vi "Set and Get Cell ItemName.vi"(6 "Cell":T1 caption="活动单元格:活动单元格", 7 "Mode":T2, 8 "错误输入":errorcluster, 10 "Item In":string, 11 "Mlistbox Ref":refnum<vi>) -> (0 "错误输出":errorcluster, 2 "Item Out":string, 3 "Mlistbox Ref Dup":refnum<vi>)   [LabVIEW 2012, in "Mlistbox Tools.lvlib"]
uses:
  Mlistbox Tools.lvlib
  ListBox/Custom Type/Read and Write Mode.ctl
  <vilib>/Utility/miscctls.llb/LVRowAndColumnTypeDef.ctl
  Set and Get ItemNames.vi
  ListBox/Listbox Tool.lvlib
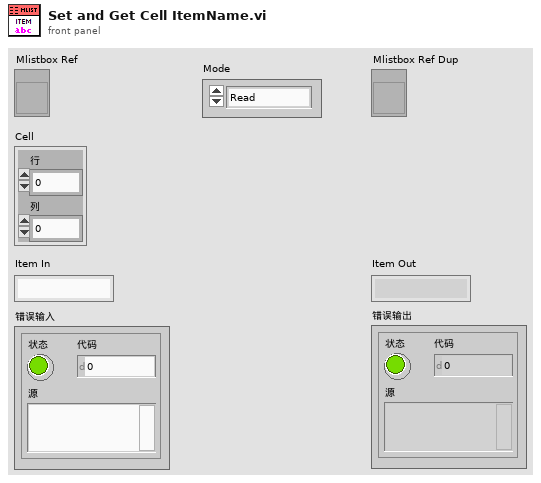
[diagram p1: front panel]
types:
  T1 = typedef "LVRowAndColumnTypeDef.ctl" = cluster{"Row":i32, "Column":i32}
  T2 = typedef "Listbox Tool.lvlib/Read and Write Mode.ctl" = enum16{"Read", "Write"}
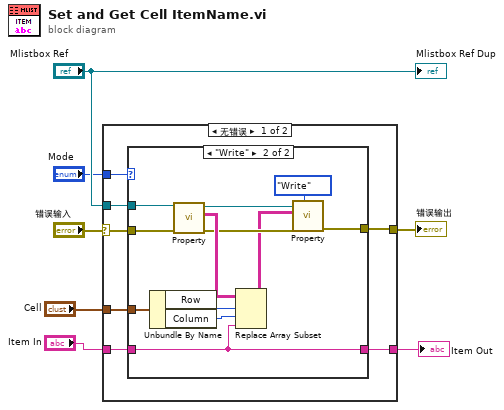
[diagram p0: block diagram]
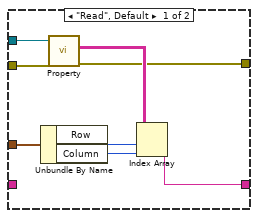
[diagram p2: hidden frame]
diagram:
  n1 = case shown="无错误" "错误输入" {
    selector: "错误输入" -> [w12 w35]
    tunnel: [w8 w35] -> w6
    tunnel: "Mlistbox Ref" -> [w13 _]
    tunnel: "Mode" -> [w14 _]
    tunnel: "Cell" -> [w11 _]
    tunnel: [w10 _] -> w1
    tunnel: "Item In" -> [w9 _]
    frame No Error {
      n2 = case shown="\"Write\"" w14 {
        tunnel: w13 -> [w18 w34]
        tunnel: w12 -> [w17 w33]
        tunnel: w11 -> [w22 w31]
        tunnel: [w19 w23] -> w10
        tunnel: w9 -> [_ w23]
        tunnel: [w15 w24] -> w8
        frame "Read", Default {
          n3 = Unbundle By Name(w22) -> ("Row"=w21:i32, "Column"=w20:i32)
          n4 = call-poly "Property.vi"("错误输入"=w17, "Mlistbox Ref"=w18) -> ("错误输出"=w15:errorcluster, "ItemNames Out"=w16:string[][])  [unwired: 7 in, 1 out]
          n5 = Index Array(array=w16, index (row)=w21, index (col)=w20) -> (element=w19:string)
        }
        frame "Write" {
          n6 = Unbundle By Name(w31) -> ("Row"=w30:i32, "Column"=w29:i32)
          n7 = call-poly "Property.vi"("错误输入"=w33, "Mlistbox Ref"=w34) -> ("错误输出"=w28:errorcluster, "ItemNames Out"=w32:string[][], "Mlistbox Ref Dup"=w27:refnum<vi>)  [unwired: 7 in]
          n8 = Replace Array Subset(array=w32, new element=w23, index (row)=w30, index (col)=w29) -> (w25:string[][])
          n9 = call-poly "Property.vi"("Mode"=Read_and_Write_Mode."Write", "错误输入"=w28, "ItemNames In"=w25, "Mlistbox Ref"=w27) -> ("错误输出"=w24:errorcluster)  [unwired: 5 in, 2 out]
        }
      }
    }
    frame Error {
    }
  }
  "错误输出" <- w6
  "Item Out" <- w1
  "Mlistbox Ref Dup" <- "Mlistbox Ref"
